vi "header_find_and_replace.vi"(9 "new value":string, 10 "field":string caption="Input Field: do not include \":\" but note that this will be expected at the end of the firld within the \"start_data_file\" VI.", 11 "text in":string) -> (0 "Exactly one match?":bool, 3 "text out":string)   [LabVIEW 2010]
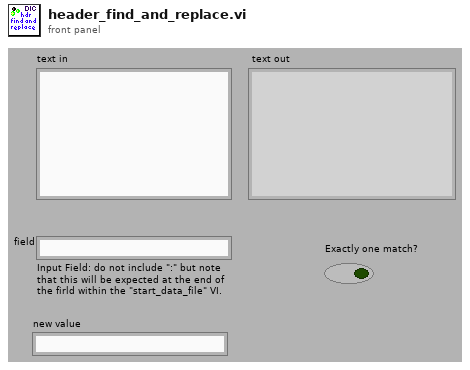
[diagram p1: front panel]
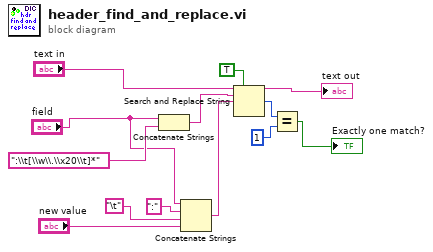
[diagram p0: block diagram]
diagram:
  n1 = Concatenate Strings("field", ":\\t[\\w\\.\\x20\\t]*") -> (w9:string)
  n2 = Concatenate Strings("field", ":", "\t", "new value") -> (w7:string)
  n3 = Search and Replace String(replace all?=TRUE, input string="text in", search string=w9, replace string=w7) -> (result string=→"text out":string, number of replacements=w5:i32)  [unwired: 4 in, 2 out]
  n4 = Equal?(x=w5, y=1) -> (x = y?=→"Exactly one match?":bool)
